vi "load_panel.vi"() -> ()   [LabVIEW 2018]
panel:
  in  "字符串":string
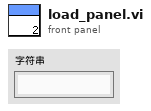
[diagram p1: front panel]
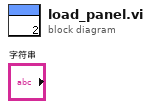
[diagram p0: block diagram]
diagram:
